vi "WLC Fitting_Final_YCC.vi"() -> ()   [LabVIEW 2014]
uses:
  <vilib>/gmath/NI_Gmath.lvlib
  <vilib>/gmath/NumericalOptimization/Nonlinear Curve Fit LM formula string.vi
  <vilib>/Utility/file.llb/Write To Spreadsheet File (DBL).vi
  <vilib>/Utility/file.llb/Read From Spreadsheet File (DBL).vi
  SubVI/WLC-Fitting Cluster.ctl
panel:
  out "Cut-Force for eWLC (pN)":dbl[](array[numeric])
  out "best nonlinear fit extension":dbl[](array[numeric])
  in  "T=use stuckbead 7th order\nF=use slope 1st order calibrate":bool=TRUE
  out "Force to be saved":dbl[](array[numeric])
  out "xDNA to be saved":dbl[](array[numeric])
  in  "T=Fit U or twoside\nF=Fit F":bool=TRUE
  out "F-Force":dbl[](array[numeric])
  out "F-xDNA":dbl[](array[numeric])
  in  "F-yr shift (mV)":dbl
  in  "F-cr shift (nm)":dbl
  out "F-QPD signal (V)":dbl[](array[numeric])
  out "F-Stage Positions (um)":dbl[](array[numeric])
  in  "stuckbead path (dialog if empty)":path=path "D:/YCC/QPD scan file/可用/x-120mW-4.txt"
  in  "F+U data?":bool
  in  "Ready to Fit":bool
  out "Save to Path":path
  out "best nonlinear fit force":dbl[](array[numeric])
  in  "SaveName":enum16{"ForecExtension Only", "WLC Fitting"}(ring)
  in  "Save Calibrated Data?":bool
  in  "Finish Fitting":bool
  out "best fit parameters":dbl[](array[numeric])
  in  "initial parameters":dbl[](array[numeric])=[40.0, 1150.0]
  in  "Enum":T1(ring)
  in  "initial parameters for fit K\n(three parameters)":dbl[](array[numeric])=[40.0, 1150.0, 1000.0]
  out "U-Force or twoside":dbl[](array[numeric])
  out "U-xDNA or twoside":dbl[](array[numeric])
  out "Fitting Cluster for indicator":T2={"cr (um)"=0.0, "yr (V)"=0.0, "trap height(nm)"=0.0, "bead radius(nm)"=520.0, "Length offset"=0.0, "Upper Force(pN)"=0.0, "cr shift (nm)"=0.0, "yr shift (mV)"=0.0, "LaserPower (mW)"=0.0, "conversion factor (V/um)"=0.0, "Stiffness (pN/nm)"=0.0154, "xDNA cut outside"=3000.0, "Lower Force(pN)"=5.0}
  in  "OneDirectionOnly?":bool=TRUE
  in  "Fitting Cluster for contorl":T3={"cr (um)"=0.0, "yr (V)"=0.0, "trap height(nm)"=300.0, "bead radius(nm)"=515.0, "Length offset"=400.0, "conversion factor (V/um)"=0.0, "Force constant (pN/nm)"=0.0154, "Force offset"=5.0, "cr shift (nm)"=0.0, "yr shift (mV)"=0.0, "LaserPower (mW)"=20.0, "Cf. Calib. Array"=[0.10641, -0.29934], "Stiffness Calib. array"=[0.0034, -0.00514]}
  in  "Tab Control":T4(tab)
  out "Stage-QPD Graph":T5(graph)
  out "U-Extension-Force Graph":cluster{"xDNA":dbl[], "Force":dbl[]}(graph)
  out "F-Extension-Force Graph":cluster{"xDNA":dbl[], "Force":dbl[]}(graph)
  out "All-Extension-Force Graph":T6(graph)
  out "Extension-Force and WLC Graph":cluster{"xDNA":dbl[], "Force":dbl[]}[](graph)
  out "Cut Stage Position (um)":dbl[](array[numeric])
  out "Cut QPD (V)":dbl[](array[numeric])
  in  "Delete Outside Signal?":bool
  out "U-QPD signal or All QPD  (V)":dbl[](array[numeric])
  out "U-Stage Positions or All stage positions (um)":dbl[](array[numeric])
  in  "Load Stage-QPD data":path
  in  "QPD":dbl[](array[numeric])
  in  "Stage":dbl[](array[numeric])
  in  "T=Read data mode?\nF=Real time fit":bool=TRUE
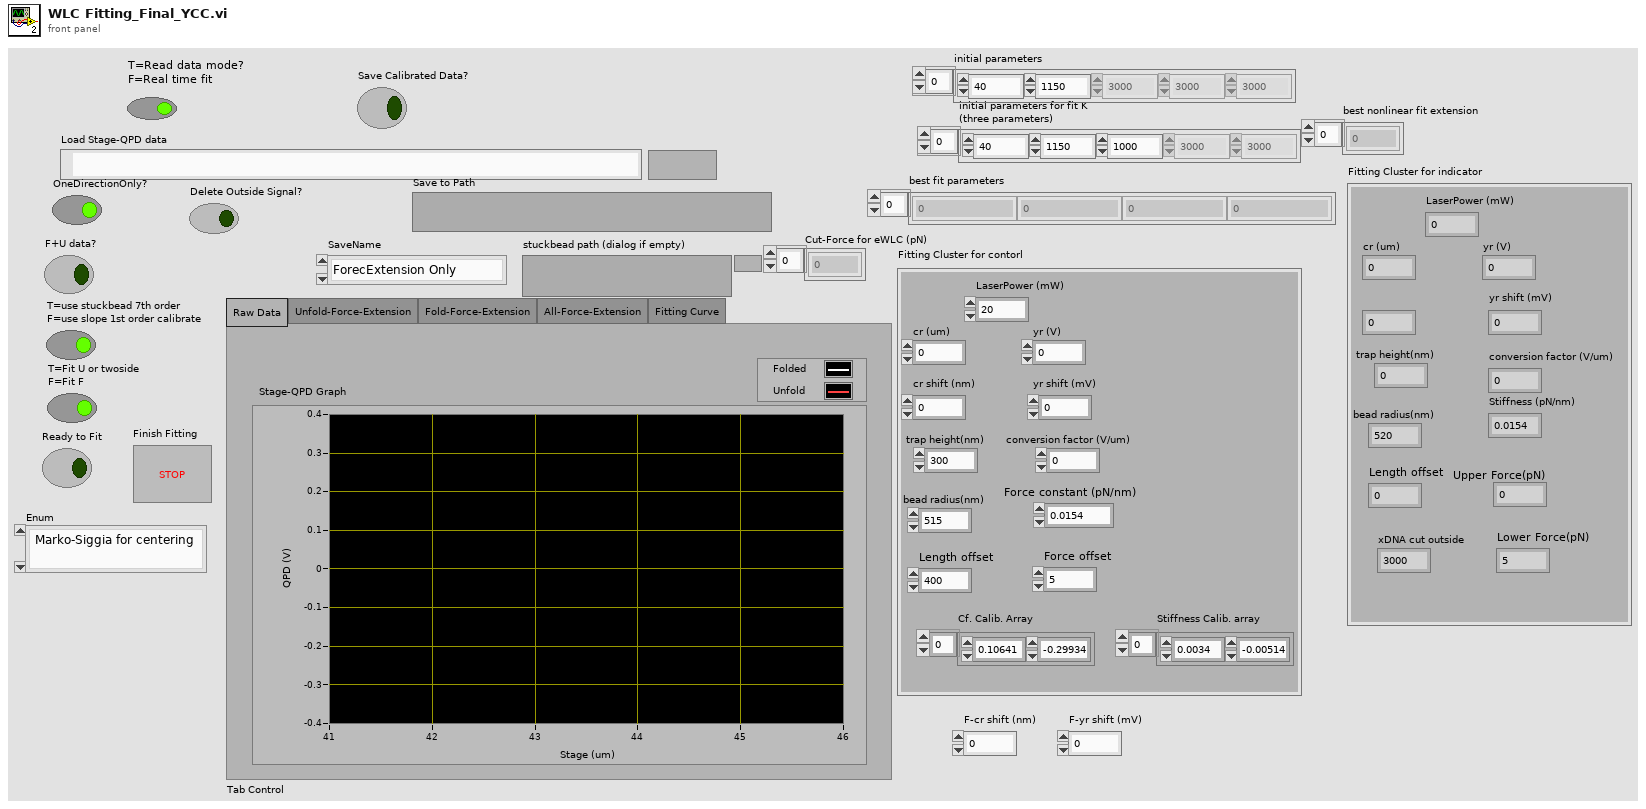
[diagram p1: front panel]
types:
  T1 = enum16{" Marko-Siggia for centering", "Marko-Siggia", "fit K (Lc,K)", "modified Marko", "eWLC (Lc,K)", "eWLC-modified M-S", "K fit eWLC-modified M-S"}
  T2 = typedef "WLC-Fitting Cluster.ctl" = cluster{"cr (um)":dbl, "yr (V)":dbl, "trap height(nm)":dbl, "bead radius(nm)":dbl, "Length offset":dbl, "Upper Force(pN)":dbl, "cr shift (nm)":dbl, "yr shift (mV)":dbl, "LaserPower (mW)":dbl, "conversion factor (V/um)":dbl, "Stiffness (pN/nm)":dbl, "xDNA cut outside":dbl, "Lower Force(pN)":dbl}
  T3 = typedef "WLC-Fitting Cluster.ctl" = cluster{"cr (um)":dbl, "yr (V)":dbl, "trap height(nm)":dbl, "bead radius(nm)":dbl, "Length offset":dbl, "conversion factor (V/um)":dbl, "Force constant (pN/nm)":dbl, "Force offset":dbl, "cr shift (nm)":dbl, "yr shift (mV)":dbl, "LaserPower (mW)":dbl, "Cf. Calib. Array":dbl[], "Stiffness Calib. array":dbl[]}
  T4 = enum32{"Raw Data", "Unfold-Force-Extension", "Fold-Force-Extension", "All-Force-Extension", "Fitting Curve"}
  T5 = cluster{"Sorted Stage Position (um)":dbl[], "Sorted QPD (V)":dbl[]}[]
  T6 = cluster{"Folded-xDNA":dbl[], "Folded-Force":dbl[]}[]
  T7 = cluster{"model":string, "Parameters":string[], "x":string}
  T8 = cluster{"F-Stage Positions (um) ":dbl[], "F-QPD signal (V) ":dbl[]}
  T9 = cluster{"U-Stage Positions or All stage positions (um)":dbl[], "U-QPD signal or All QPD  (V)":dbl[]}
  T10 = cluster{"U-Stage Positions or All stage positions (um)":dbl[], "U-QPD signal or All QPD  (V)":dbl[]}[]
  T11 = cluster{"Unfolded-xDNA":dbl[], "Unfolded-Force":dbl[]}
  T12 = cluster{"Folded-xDNA":dbl[], "Folded-Force":dbl[]}
  T13 = cluster{"Unfolded-xDNA":dbl[], "Unfolded-Force":dbl[]}[]
  T14 = cluster{"U-xDNA or twoside":dbl[], "best nonlinear fit":dbl[]}
  T15 = cluster{"U-xDNA or twoside":dbl[], "U-Force or twoside":dbl[]}
  T16 = cluster{"best nonlinear fit extension for eWLC":dbl[], "Cut-Force (pN)":dbl[]}
  T17 = cluster{"best nonlinear fit extension for eWLC":dbl[], "Cut-Force (pN)":dbl[]}[]
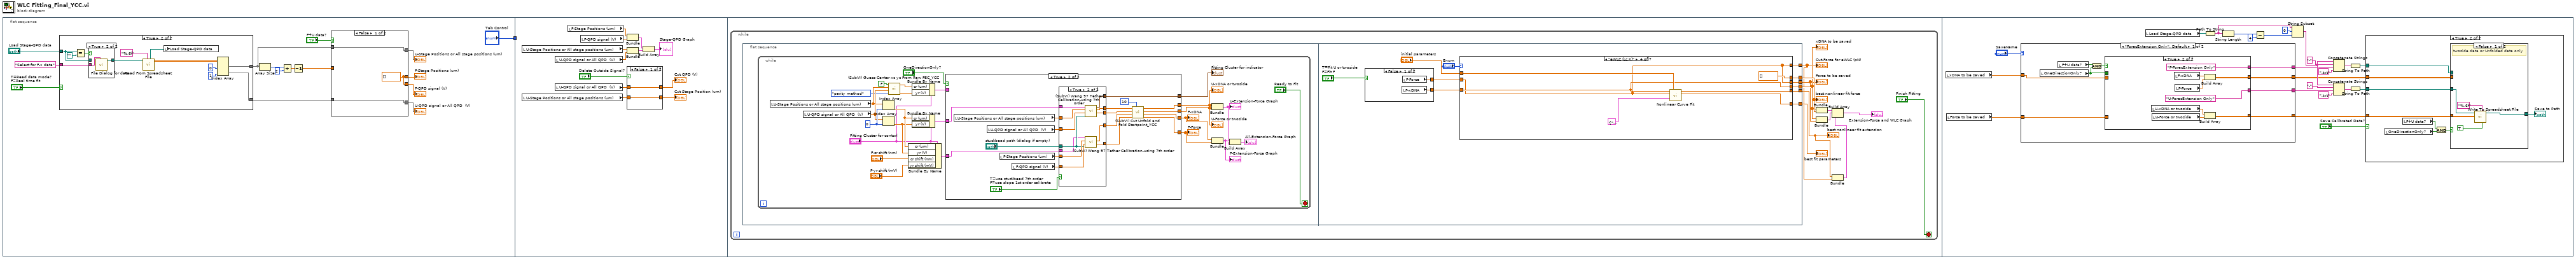
[diagram p0: block diagram]
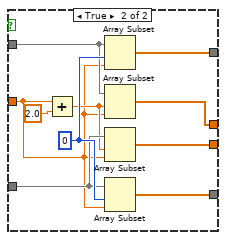
[diagram p2: hidden frame]
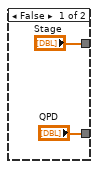
[diagram p3: hidden frame]
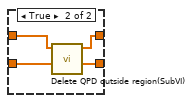
[diagram p5: hidden frame]
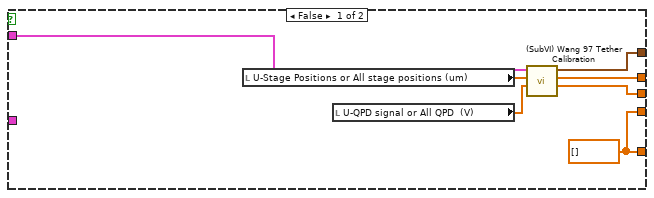
[diagram p6: hidden frame]
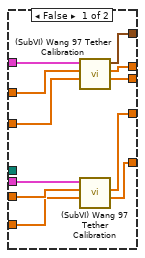
[diagram p7: hidden frame]
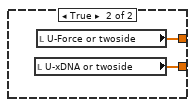
[diagram p8: hidden frame]
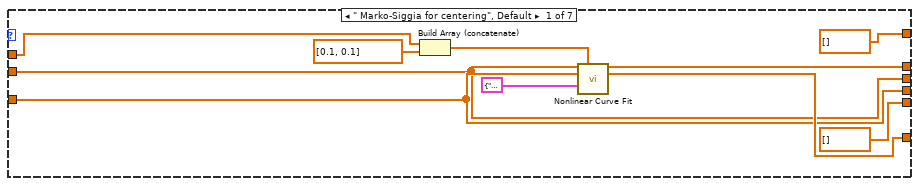
[diagram p9: hidden frame]
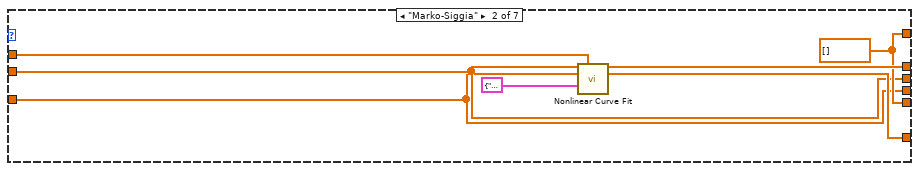
[diagram p10: hidden frame]
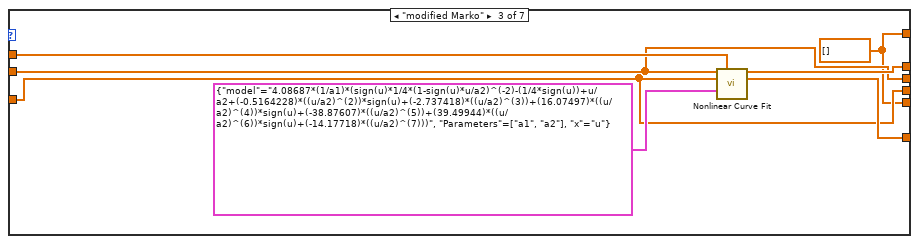
[diagram p11: hidden frame]
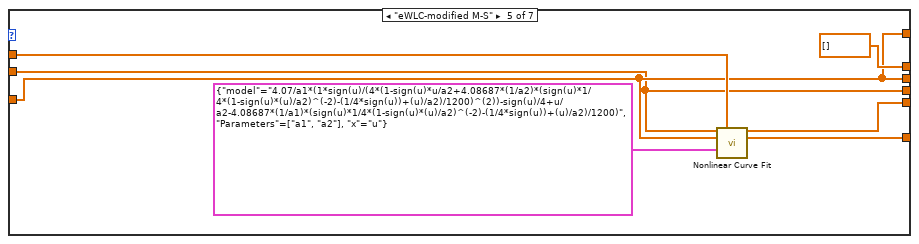
[diagram p12: hidden frame]
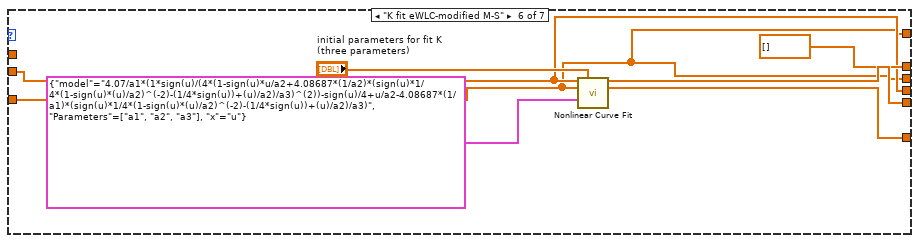
[diagram p13: hidden frame]
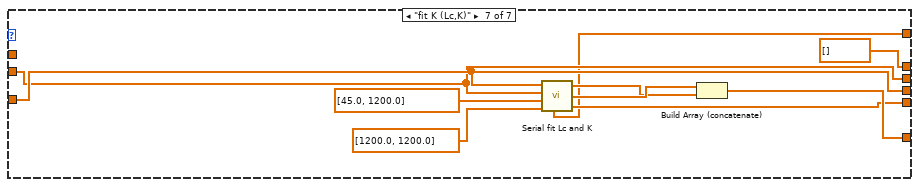
[diagram p14: hidden frame]
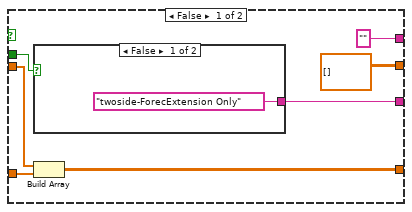
[diagram p15: hidden frame]
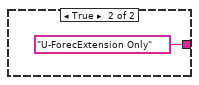
[diagram p16: hidden frame]
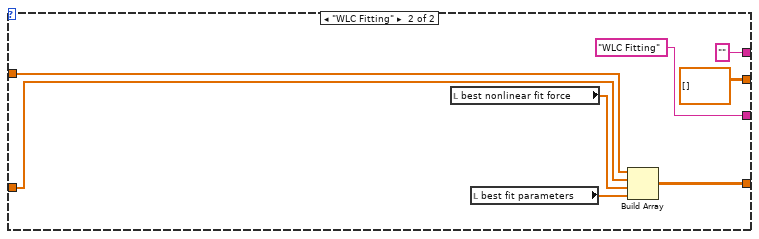
[diagram p17: hidden frame]
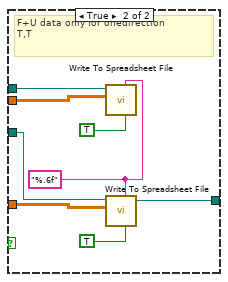
[diagram p19: hidden frame]
diagram:
  n1 = flat-sequence {
    tunnel: ["Tab Control"] -> w1
    tunnel: w1 -> [_]
    frame #0 {
      n2 = case shown="True" "T=Read data mode?\nF=Real time fit" {
        tunnel: ["QPD" w39] -> w11
        tunnel: ["Stage" w40] -> w6
        tunnel: "Select for F-x data" ("default name") -> [_ w36]
        tunnel: "Load Stage-QPD data" -> [_ w33]
        frame False {
        }
        frame True {
          n3 = Equal?(x=w33, y=path "") -> (x = y?=w34:bool)
          n4 = case shown="True" w34 {
            tunnel: [w44 w45] -> w37
            tunnel: w36 -> [_ w46]
            tunnel: w33 -> [w44 _]
            frame False {
            }
            frame True {
              n5 = call "File Dialog for data"("prompt"=w46) -> ("selected path"=w45:path)  [unwired: 11 in, 3 out]
            }
          }
          n6 = call-poly <vilib>:"Read From Spreadsheet File.vi"("format (%.3f)"="%.6f", "file path (dialog if empty)"=w37) -> ("all rows"=w43:dbl[][], "new file path (Not A Path if cancelled)"=w32:path)  [unwired: 5 in, 3 out]
          n7 = local write "Load Stage-QPD data"(w32) -> ()
          n8 = Index Array(array=w43, index (col) #1=0 ("disabled index (col)"), index (col) #2=1 ("index (col)")) -> (element #1=w40:dbl[], element #2=w39:dbl[])  [unwired: 2 in]
        }
      }
      n9 = Array Size(array=w6) -> (size(s)=w7:i32)
      n10 = Divide(x=w7, y=2) -> (x/y=w5:dbl)
      n11 = Decrement(x=w5) -> (x-1=w4:dbl)
      n12 = case shown="False" "F+U data?" {
        tunnel: w6 -> [w19 w25]
        tunnel: w11 -> [w18 w26]
        tunnel: [w19 w29] -> w10
        tunnel: [w18 w27] -> w9
        tunnel: w4 -> [_ w20]
        tunnel: [w17 w24] -> w3
        tunnel: [w17 w23] -> w2
        frame False {
          w17 = dbl[] []
        }
        frame True {
          w28 = 0 ("index")
          n13 = Add(x=w20, y=2.0) -> (x+y=w21:dbl)
          n14 = Array Subset(array=w25, index=w28, length=w20) -> (w29:dbl[])
          n15 = Array Subset(array=w25, index=w21, length=w20) -> (w24:dbl[])
          n16 = Array Subset(array=w26, index=w21, length=w20) -> (w23:dbl[])
          n17 = Array Subset(array=w26, index=w28, length=w20) -> (w27:dbl[])
        }
      }
      "U-Stage Positions or All stage positions (um)" <- w10
      "U-QPD signal or All QPD  (V)" <- w9
      "F-Stage Positions (um)" <- w3
      "F-QPD signal (V)" <- w2
    }
    frame #1 {
      n18 = local read "U-Stage Positions or All stage positions (um)"() -> (w55:dbl[])
      n19 = local read "U-Stage Positions or All stage positions (um)"() -> (w57:dbl[])
      n20 = local read "U-QPD signal or All QPD  (V)"() -> (w54:dbl[])
      n21 = local read "U-QPD signal or All QPD  (V)"() -> (w56:dbl[])
      n22 = local read "F-Stage Positions (um)"() -> (w48:dbl[])
      n23 = local read "F-QPD signal (V)"() -> (w47:dbl[])
      n24 = Bundle("F-Stage Positions (um)"=w48, "F-QPD signal (V)"=w47) -> (w53:T8)  [unwired: 1 in]
      n25 = Bundle("U-Stage Positions or All stage positions (um)"=w55, "U-QPD signal or All QPD  (V)"=w54) -> (w52:T9)  [unwired: 1 in]
      n26 = case shown="False" "Delete Outside Signal?" {
        tunnel: w56 -> [w60 w64]
        tunnel: w57 -> [w59 w63]
        tunnel: [w60 w62] -> w49
        tunnel: [w59 w61] -> w50
        frame False {
        }
        frame True {
          n27 = call "Delete QPD outside region(SubVI).vi"("Position Array In"=w63, "QPD signal In"=w64) -> ("Position Array Out"=w61:dbl[], "QPD signal Out"=w62:dbl[])  [unwired: 8 in]
        }
      }
      "Cut QPD (V)" <- w49
      "Cut Stage Position (um)" <- w50
      n28 = Build Array(w53, w52) -> (→"Stage-QPD Graph":T10)
    }
    frame #2 {
      n29 = while {
        stop <- "Finish Fitting" stop-if-true
        n30 = flat-sequence {
          tunnel: [w157] -> w71
          tunnel: [w156] -> w70
          tunnel: [w152] -> w69
          tunnel: [w151] -> w68
          tunnel: [w150] -> w67
          tunnel: [w149] -> w66
          frame #0 {
            n31 = while {
              stop <- "Ready to Fit" stop-if-true
              w99 = 0 ("index")
              n32 = local read "U-Stage Positions or All stage positions (um)"() -> (w86:dbl[])
              n33 = local read "U-QPD signal or All QPD  (V)"() -> (w85:dbl[])
              n34 = Index Array(array=w86, index=w99) -> (element=w95:dbl)
              n35 = Index Array(array=w85, index=w99) -> (element=w94:dbl)
              n36 = call "(SubVI) Guess Center xc yc From Raw FEC_YCC.vi"("Enum"=enum16{"parity method", "max-min method"}."parity method", "QPD array (V)"=w85, "Stage array(um)"=w86, "Read data?"=FALSE) -> ("Guess-QPD-center (V)"=w83:dbl, "Guess-stage-center (um)"=w84:dbl)  [unwired: 1 in]
              n37 = Bundle By Name(cluster="Fitting Cluster for contorl", "cr (um)"=w95, "yr (V)"=w94, "cr shift (nm)"="F-cr shift (nm)", "yr shift (mV)"="F-yr shift (mV)") -> (w91:T3)
              n38 = Bundle By Name(cluster="Fitting Cluster for contorl", "cr (um)"=w84, "yr (V)"=w83) -> (w82:T3)
              n39 = Bundle By Name(cluster="Fitting Cluster for contorl", "cr (um)"=w95, "yr (V)"=w94) -> (w98:T3)
              n40 = case shown="True" "OneDirectionOnly?" {
                tunnel: w98 -> [_ w123]
                tunnel: [w104 w124] -> w97
                tunnel: w91 -> [_ w118]
                tunnel: w82 -> [w107 _]
                tunnel: [w103 w112] -> w81
                tunnel: [w102 w111] -> w80
                tunnel: [w101 w110] -> w79
                tunnel: [w101 w109] -> w78
                frame False {
                  w101 = dbl[] [] ("Folded-xDNA")
                  n41 = local read "U-Stage Positions or All stage positions (um)"() -> (w106:dbl[])
                  n42 = local read "U-QPD signal or All QPD  (V)"() -> (w105:dbl[])
                  n43 = call "(SubVI) Wang 97 Tether Calibration.vi"("QPD signal"=w105, "Stage Position"=w106, "Fitting Cluster"=w107) -> ("Force"=w102:dbl[], "xDNA"=w103:dbl[], "output cluster"=w104:T2)  [unwired: 2 in]
                }
                frame True {
                  n44 = local read "U-Stage Positions or All stage positions (um)"() -> (w122:dbl[])
                  n45 = local read "U-QPD signal or All QPD  (V)"() -> (w125:dbl[])
                  n46 = local read "F-Stage Positions (um)"() -> (w121:dbl[])
                  n47 = local read "F-QPD signal (V)"() -> (w120:dbl[])
                  n48 = case shown="True" "T=use stuckbead 7th order\nF=use slope 1st order calibrate" {
                    tunnel: w125 -> [w134 w148]
                    tunnel: [w133 w147] -> w124
                    tunnel: w123 -> [w136 w146]
                    tunnel: w122 -> [w135 w145]
                    tunnel: w121 -> [w131 w144]
                    tunnel: w120 -> [w130 w143]
                    tunnel: "stuckbead path (dialog if empty)" -> [_ w142]
                    tunnel: w118 -> [w132 w141]
                    tunnel: [w129 w140] -> w116
                    tunnel: [w128 w139] -> w115
                    tunnel: [w127 w138] -> w114
                    tunnel: [w126 w137] -> w113
                    frame False {
                      n49 = call "(SubVI) Wang 97 Tether Calibration.vi"("QPD signal"=w134, "Stage Position"=w135, "Fitting Cluster"=w136) -> ("Force"=w128:dbl[], "xDNA"=w129:dbl[], "output cluster"=w133:T2)  [unwired: 2 in]
                      n50 = call "(SubVI) Wang 97 Tether Calibration.vi"("QPD signal"=w130, "Stage Position"=w131, "Fitting Cluster"=w132) -> ("Force"=w126:dbl[], "xDNA"=w127:dbl[])  [unwired: 2 in, 1 out]
                    }
                    frame True {
                      n51 = call "(SubVI) Wang 97 Tether Calibration-using 7th order.vi"("stuckbead path (dialog if empty)"=w142, "QPD signal"=w148, "Stage Position"=w145, "Fitting Cluster"=w146) -> ("Force"=w139:dbl[], "xDNA"=w140:dbl[], "output cluster"=w147:T2)  [unwired: 3 in, 2 out]
                      n52 = call "(SubVI) Wang 97 Tether Calibration-using 7th order.vi"("stuckbead path (dialog if empty)"=w142, "QPD signal"=w143, "Stage Position"=w144, "Fitting Cluster"=w141) -> ("Force"=w137:dbl[], "xDNA"=w138:dbl[])  [unwired: 3 in, 3 out]
                    }
                  }
                  n53 = call "(SubVI) Cut Unfold and Fold Startpoint_YCC.vi"("number to cut"=10, "Folded-Force in"=w113, "Folded-xDNA in"=w114, "Unfolded-Force"=w115, "Unfolded-xDNA"=w116) -> ("Folded-Force"=w109:dbl[], "Folded-xDNA"=w110:dbl[], "Unfolded-Force"=w111:dbl[], "Unfolded-xDNA"=w112:dbl[])  [unwired: 3 in]
                }
              }
              "Fitting Cluster for indicator" <- w97
              "U-xDNA or twoside" <- w81
              "U-Force or twoside" <- w80
              "F-xDNA" <- w79
              "F-Force" <- w78
              n54 = Bundle("Unfolded-xDNA"=w81, "Unfolded-Force"=w80) -> (w88:T11)  [unwired: 1 in]
              "U-Extension-Force Graph" <- w88
              n55 = Bundle("Folded-xDNA"=w79, "Folded-Force"=w78) -> (w89:T12)  [unwired: 1 in]
              "F-Extension-Force Graph" <- w89
              n56 = Build Array(w89, w88) -> (→"All-Extension-Force Graph":T13)
            }
          }
          frame #1 {
            n57 = case shown="False" "T=Fit U or twoside\nF=Fit F" {
              tunnel: [w161 w163] -> w155
              tunnel: [w160 w162] -> w154
              frame False {
                n58 = local read "F-xDNA"() -> (w161:dbl[])
                n59 = local read "F-Force"() -> (w160:dbl[])
              }
              frame True {
                n60 = local read "U-xDNA or twoside"() -> (w163:dbl[])
                n61 = local read "U-Force or twoside"() -> (w162:dbl[])
              }
            }
            n62 = case shown="\"eWLC (Lc,K)\"" "Enum" {
              tunnel: "initial parameters" -> [w170 w177 w186 w193 w200 _ _]
              tunnel: w154 -> [w164 w175 w183 w188 w195 w203 w214]
              tunnel: w155 -> [w165 w174 w182 w189 w196 w202 w215]
              tunnel: [w168 w179 w184 dbl[] [] ("best nonlinear fit") dbl[] [] ("best nonlinear fit") dbl[] [] ("best nonlinear fit") dbl[] [] ("best nonlinear fit")] -> w157
              tunnel: [w169 w178 w185 w192 w199 w206 w216] -> w156
              tunnel: [w165 w174 w182 w189 w195 w203 w215] -> w152
              tunnel: [w164 w175 w183 w188 w196 w202 w214] -> w151
              tunnel: [dbl[] [] ("best nonlinear fit extension for eWLC") w176 w181 w191 w198 w205 w211] -> w150
              tunnel: [dbl[] [] ("Cut-Force (pN)") w176 w181 w188 w196 w202 w209] -> w149
              frame " Marko-Siggia for centering", Default {
                n63 = Build Array (concatenate)(w170, dbl[] [0.1, 0.1] ("element")) -> (w171:dbl[])
                n64 = call-poly <vilib>:"Nonlinear Curve Fit.vi"("Y"=w164, "initial parameters"=w171, "X"=w165, "model description"=T7 {"model"="4.08687*(1/a1)*(sign(u-a3)*1/4*(1-sign(u-a3)*(u-a3)/a2)^(-2)-(1/4*sign(u-a3))+(u-a3)/a2)+a4", "Parameters"=["a1", "a2", "a3", "a4"], "x"="u"}) -> ("best nonlinear fit"=w168:dbl[], "best fit parameters"=w169:dbl[])  [unwired: 3 in, 7 out]
              }
              frame "Marko-Siggia" {
                w176 = dbl[] [] ("best nonlinear fit extension for eWLC")
                n65 = call-poly <vilib>:"Nonlinear Curve Fit.vi"("Y"=w175, "initial parameters"=w177, "X"=w174, "model description"=T7 {"model"="4.08687*(1/a1)*(sign(u)*1/4*(1-sign(u)*u/a2)^(-2)-(1/4*sign(u))+u/a2)", "Parameters"=["a1", "a2"], "x"="u"}) -> ("best nonlinear fit"=w179:dbl[], "best fit parameters"=w178:dbl[])  [unwired: 3 in, 7 out]
              }
              frame "modified Marko" {
                w181 = dbl[] [] ("best nonlinear fit extension for eWLC")
                n66 = call-poly <vilib>:"Nonlinear Curve Fit.vi"("Y"=w183, "initial parameters"=w186, "X"=w182, "model description"=T7 {"model"="4.08687*(1/a1)*(sign(u)*1/4*(1-sign(u)*u/a2)^(-2)-(1/4*sign(u))+u/a2+(-0.5164228)*((u/a2)^(2))*sign(u)+(-2.737418)*((u/a2)^(3))+(16.07497)*((u/a2)^(4))*sign(u)+(-38.87607)*((u/a2)^(5))+(39.49944)*((u/a2)^(6))*sign(u)+(-14.17718)*((u/a2)^(7)))", "Parameters"=["a1", "a2"], "x"="u"}) -> ("best nonlinear fit"=w184:dbl[], "best fit parameters"=w185:dbl[])  [unwired: 3 in, 7 out]
              }
              frame "eWLC (Lc,K)" {
                n67 = call-poly <vilib>:"Nonlinear Curve Fit.vi"("Y"=w189, "initial parameters"=w193, "X"=w188, "model description"=T7 {"model"="a1*(1*sign(u)-sign(u)*1/2*(4.07/u/45)^(0.5)+sign(u)*u/a2)", "Parameters"=["a1", "a2"], "x"="u"}) -> ("best nonlinear fit"=w191:dbl[], "best fit parameters"=w192:dbl[])  [unwired: 3 in, 7 out]
              }
              frame "eWLC-modified M-S" {
                n68 = call-poly <vilib>:"Nonlinear Curve Fit.vi"("Y"=w195, "initial parameters"=w200, "X"=w196, "model description"=T7 {"model"="4.07/a1*(1*sign(u)/(4*(1-sign(u)*u/a2+4.08687*(1/a2)*(sign(u)*1/4*(1-sign(u)*(u)/a2)^(-2)-(1/4*sign(u))+(u)/a2)/1200)^(2))-sign(u)/4+u/a2-4.08687*(1/a1)*(sign(u)*1/4*(1-sign(u)*(u)/a2)^(-2)-(1/4*sign(u))+(u)/a2)/1200)", "Parameters"=["a1", "a2"], "x"="u"}) -> ("best nonlinear fit"=w198:dbl[], "best fit parameters"=w199:dbl[])  [unwired: 7 in, 3 out]
              }
              frame "K fit eWLC-modified M-S" {
                n69 = call-poly <vilib>:"Nonlinear Curve Fit.vi"("Y"=w203, "initial parameters"="initial parameters for fit K\n(three parameters)", "X"=w202, "model description"=T7 {"model"="4.07/a1*(1*sign(u)/(4*(1-sign(u)*u/a2+4.08687*(1/a2)*(sign(u)*1/4*(1-sign(u)*(u)/a2)^(-2)-(1/4*sign(u))+(u)/a2)/a3)^(2))-sign(u)/4+u/a2-4.08687*(1/a1)*(sign(u)*1/4*(1-sign(u)*(u)/a2)^(-2)-(1/4*sign(u))+(u)/a2)/a3)", "Parameters"=["a1", "a2", "a3"], "x"="u"}) -> ("best nonlinear fit"=w205:dbl[], "best fit parameters"=w206:dbl[])  [unwired: 7 in, 3 out]
              }
              frame "fit K (Lc,K)" {
                n70 = call "Serial fit Lc and K.vi"("Extension (nm)"=w215, "Force (pN)"=w214, "initial parameters for WLC (Lp,Lc)"=dbl[] [45.0, 1200.0], "initial parameters for eWLC (Lc,K)"=dbl[] [1200.0, 1200.0]) -> ("Cut-Force (pN)"=w209:dbl[], "best fit parameters for eWLC (Lp,Lc,K)"=w212:dbl[], "best fit parameters for WLC"=w213:dbl[], "best nonlinear fit extension for eWLC"=w211:dbl[])  [unwired: 1 out]
                n71 = Build Array (concatenate)(w213, w212) -> (w216:dbl[])
              }
            }
          }
        }
        n72 = Bundle("U-xDNA or twoside"=w69, "best nonlinear fit"=w71) -> (w74:T14)  [unwired: 1 in]
        n73 = Bundle("U-xDNA or twoside"=w69, "U-Force or twoside"=w68) -> (w73:T15)  [unwired: 1 in]
        n74 = Bundle("best nonlinear fit extension for eWLC"=w67, "Cut-Force (pN)"=w66) -> (w65:T16)  [unwired: 1 in]
        n75 = Build Array(w74, w73, w65) -> (→"Extension-Force and WLC Graph":T17)
        "best nonlinear fit force" <- w71
        "best fit parameters" <- w70
        "xDNA to be saved" <- w69
        "Force to be saved" <- w68
        "best nonlinear fit extension" <- w67
        "Cut-Force for eWLC (pN)" <- w66
      }
    }
    frame #3 {
      n76 = local read "xDNA to be saved"() -> (w220:dbl[])
      n77 = local read "Force to be saved"() -> (w219:dbl[])
      n78 = case shown="\"ForecExtension Only\", Default" "SaveName" {
        tunnel: [w250 "WLC Fitting" ("string")] -> w232
        tunnel: [w249 w272] -> w229
        tunnel: [w248 "" ("string")] -> w224
        tunnel: [w247 dbl[][] []] -> w221
        tunnel: w220 -> [w244 w269]
        tunnel: w219 -> [w243 w268]
        frame "ForecExtension Only", Default {
          n79 = local read "OneDirectionOnly?"() -> (w242:bool)
          n80 = local read "F+U data?"() -> (w246:bool)
          n81 = And(x=w246, y=w242) -> (x .and. y?=w245:bool)
          n82 = case shown="True" w245 {
            tunnel: [w257 "U-ForecExtension Only" ("string")] -> w250
            tunnel: [w254 w264] -> w249
            tunnel: ["" ("string") "F-ForecExtension Only" ("string")] -> w248
            tunnel: [dbl[][] [] w260] -> w247
            tunnel: w244 -> [w253 _]
            tunnel: w243 -> [w252 _]
            tunnel: w242 -> [w251 _]
            frame False {
              n83 = case shown="False" w251 {
                tunnel: ["twoside-ForecExtension Only" ("string") "U-ForecExtension Only" ("string")] -> w257
                frame False {
                }
                frame True {
                }
              }
              n84 = Build Array(w253, w252) -> (w254:dbl[][])
            }
            frame True {
              n85 = local read "U-xDNA or twoside"() -> (w266:dbl[])
              n86 = local read "U-Force or twoside"() -> (w265:dbl[])
              n87 = local read "F-xDNA"() -> (w263:dbl[])
              n88 = local read "F-Force"() -> (w262:dbl[])
              n89 = Build Array(w263, w262) -> (w260:dbl[][])
              n90 = Build Array(w266, w265) -> (w264:dbl[][])
            }
          }
        }
        frame "WLC Fitting" {
          n91 = local read "best nonlinear fit force"() -> (w274:dbl[])
          n92 = local read "best fit parameters"() -> (w273:dbl[])
          n93 = Build Array(w269, w268, w274, w273) -> (w272:dbl[][])
        }
      }
      n94 = local read "Load Stage-QPD data"() -> (w241:path)
      n95 = Path To String(path=w241) -> (string=w239:string)
      n96 = String Length(string=w239) -> (length=w238:i32)
      n97 = Subtract(x=w238, y=4) -> (x-y=w235:i32)
      n98 = String Subset(string=w239, offset (0)=0, length (rest)=w235) -> (substring=w226:string)
      n99 = Concatenate Strings(w226, "-" ("string"), w224, ".txt" ("string")) -> (w227:string)
      n100 = Concatenate Strings(w226, "-" ("string"), w232, ".txt" ("string")) -> (w228:string)
      n101 = String To Path(string=w227) -> (path=w222:path)
      n102 = String To Path(string=w228) -> (path=w230:path)
      n103 = case shown="True" "Save Calibrated Data?" {
        tunnel: w230 -> [_ w283]
        tunnel: w229 -> [_ w282]
        tunnel: w222 -> [_ w281]
        tunnel: w221 -> [_ w280]
        frame False {
        }
        frame True {
          n104 = local read "OneDirectionOnly?"() -> (w278:bool)
          n105 = local read "F+U data?"() -> (w277:bool)
          n106 = And(x=w277, y=w278) -> (x .and. y?=w276:bool)
          n107 = case shown="False" w276 {
            tunnel: w283 -> [w285 w296]
            tunnel: w282 -> [w286 w295]
            tunnel: w281 -> [_ w292]
            tunnel: w280 -> [_ w291]
            tunnel: [w284 w289] -> w279
            frame False {
              # "twoside data or Unfolded data only"
              n108 = call-poly <vilib>:"Write To Spreadsheet File.vi"("transpose? (no:F)"=TRUE, "format (%.3f)"="%.6f", "2D data"=w286, "file path (dialog if empty)"=w285) -> ("new file path (Not A Path if cancelled)"=w284:path)  [unwired: 4 in]
            }
            frame True {
              w293 = "%.6f" ("format (%.3f)")
              # "F+U data only for onedirection\nT,T"
              n109 = call-poly <vilib>:"Write To Spreadsheet File.vi"("transpose? (no:F)"=TRUE, "format (%.3f)"=w293, "2D data"=w291, "file path (dialog if empty)"=w292) -> ()  [unwired: 4 in, 1 out]
              n110 = call-poly <vilib>:"Write To Spreadsheet File.vi"("transpose? (no:F)"=TRUE, "format (%.3f)"=w293, "2D data"=w295, "file path (dialog if empty)"=w296) -> ("new file path (Not A Path if cancelled)"=w289:path)  [unwired: 4 in]
            }
          }
          "Save to Path" <- w279
        }
      }
    }
  }
